vi "main.vi"() -> ()   [LabVIEW 2017]
uses:
  AEROTECstageAPI/SingleStageData.ctl
  AEROTECstageAPI/StageEnum.ctl
  AEROTECstageAPI/MoveDistanceInAxis.ctl
panel:
  in  "Disable Stage":bool
  in  "Distance (mm)":dbl
  in  "Left Button":bool
  in  "Right Button":bool
  in  "Down Button":bool
  in  "Up Button":bool
  in  "Enable Stage":bool
  out "Stage Data":T1[](array[typedef])
  out "error out":errorcluster
  in  "stop 2":bool
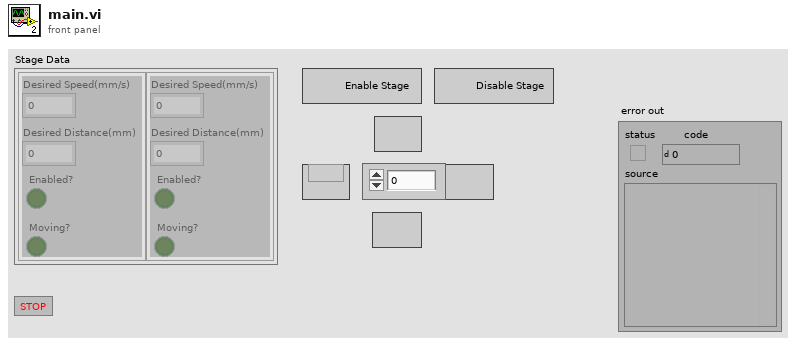
[diagram p1: front panel]
types:
  T1 = typedef "SingleStageData.ctl" = cluster{"Desired Speed(mm/s)":dbl, "Desired Distance(mm)":dbl, "Enabled?":bool, "Moving?":bool}
  T2 = typedef "StageEnum.ctl" = enum16{"Move axis!", "Enable Stage!", "Stop Stage Controller!", "Set Default Speeds!", "Get Stage Parameters", "Start Stage Controller!", "Init"}
  T3 = typedef "MoveDistanceInAxis.ctl" = cluster{"Axis Number":i16, "Distance (mm)":dbl}
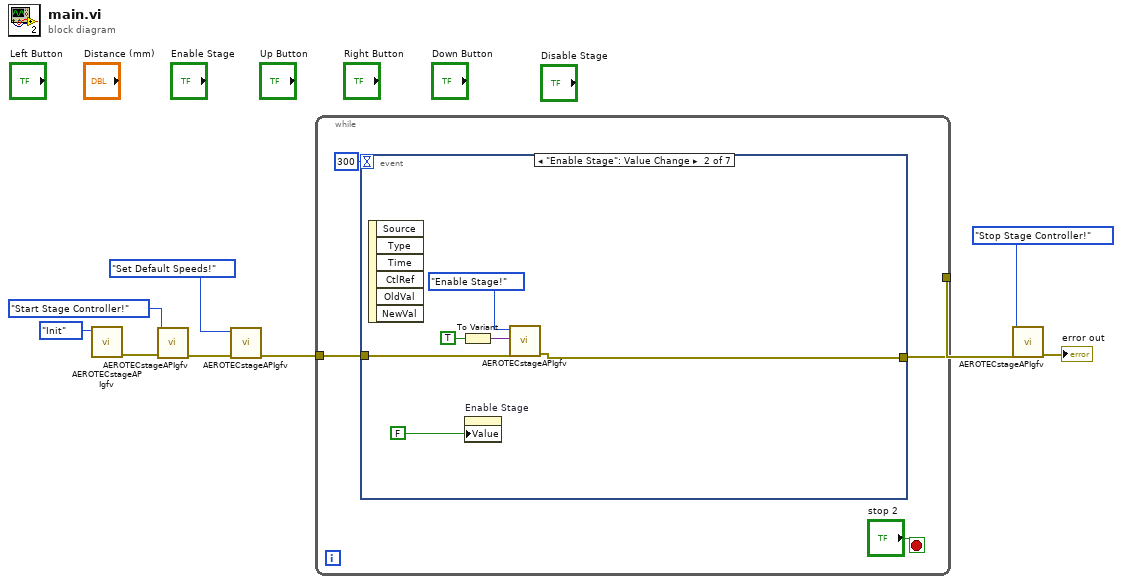
[diagram p0: block diagram]
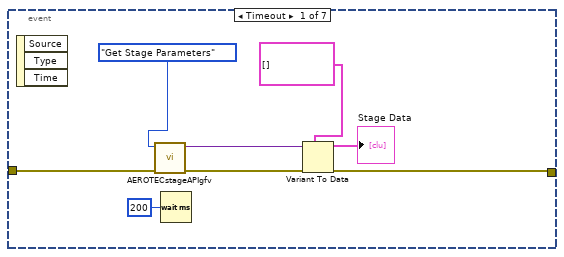
[diagram p2: hidden frame]
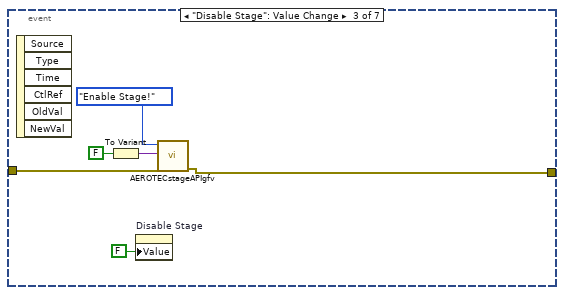
[diagram p3: hidden frame]
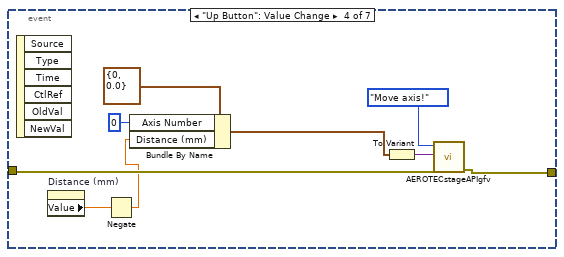
[diagram p4: hidden frame]
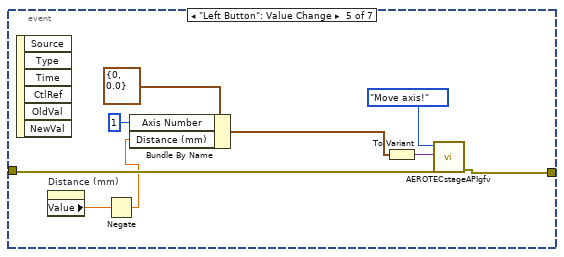
[diagram p5: hidden frame]
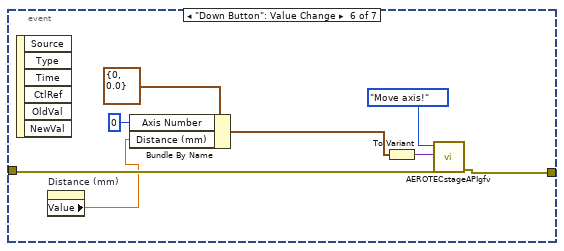
[diagram p6: hidden frame]
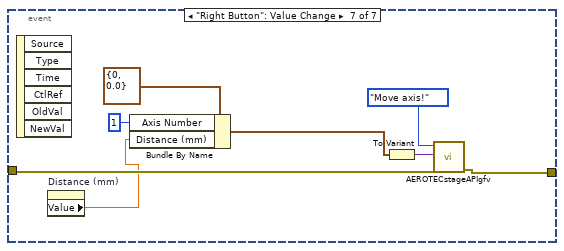
[diagram p7: hidden frame]
diagram:
  n1 = call "AEROTECstageAPIgfv.vi"(11:StageEnum."Init") -> ("error out"=w8:errorcluster)  [unwired: 9 in, 1 out]
  n2 = call "AEROTECstageAPIgfv.vi"("error in (no error)"=w8, 11:StageEnum."Start Stage Controller!") -> ("error out"=w4:errorcluster)  [unwired: 8 in, 1 out]
  n3 = call "AEROTECstageAPIgfv.vi"("error in (no error)"=w4, 11:StageEnum."Set Default Speeds!") -> ("error out"=w2:errorcluster)  [unwired: 8 in, 1 out]
  n4 = while {
    tunnel: w2 -> [w11]
    tunnel: [w10] -> w1
    stop <- "stop 2" stop-if-true
    n5 = event shown="[1] \"Enable Stage\": Value Change" {
      selector: _ -> [_ _ _ _ _ _ _]
      dyn-events: _ -> [_ _ _ _ _ _ _]
      timeout: 300 -> [_ _ _ _ _ _ _]
      tunnel: w11 -> [w16 w26 w32 w41 w50 w58 w66]
      tunnel: [w14 w25 w31 w40 w49 w57 w65] -> w10
      event Timeout {
        n6 = event-data() -> ()  [unwired: 1 in, 3 out]
        n7 = call "AEROTECstageAPIgfv.vi"("error in (no error)"=w16, 11:StageEnum."Get Stage Parameters") -> ("error out"=w14:errorcluster, "Data Out"=w20:variant)  [unwired: 8 in]
        n8 = Wait (ms)(milliseconds to wait=u32 200) -> ()  [unwired: 1 out]
        n9 = Variant To Data(type=T1[] [], Variant=w20) -> (data=→"Stage Data":T1[])  [unwired: 1 in, 1 out]
      }
      event "Enable Stage": Value Change {
        n10 = event-data() -> ()  [unwired: 1 in, 6 out]
        n11 = To Variant(anything=TRUE) -> (Variant=w22:variant)
        n12 = property on="Enable Stage" class="Bool (strict)"("Value"=FALSE) -> ()  [unwired: 2 in, 2 out]
        n13 = call "AEROTECstageAPIgfv.vi"("error in (no error)"=w26, "Data in"=w22, 11:StageEnum."Enable Stage!") -> ("error out"=w25:errorcluster)  [unwired: 7 in, 1 out]
      }
      event "Disable Stage": Value Change {
        n14 = event-data() -> ()  [unwired: 1 in, 6 out]
        n15 = To Variant(anything=FALSE) -> (Variant=w28:variant)
        n16 = property on="Disable Stage" class="Bool (strict)"("Value"=FALSE ("Disable Stage")) -> ()  [unwired: 2 in, 2 out]
        n17 = call "AEROTECstageAPIgfv.vi"("error in (no error)"=w32, "Data in"=w28, 11:StageEnum."Enable Stage!") -> ("error out"=w31:errorcluster)  [unwired: 7 in, 1 out]
      }
      event "Up Button": Value Change {
        n18 = event-data() -> ()  [unwired: 1 in, 6 out]
        n19 = property on="Distance (mm)" class="DigNum (strict)"() -> ("Value"=w34:dbl)  [unwired: 2 in, 2 out]
        n20 = Negate(x=w34) -> (-x=w33:dbl)
        n21 = Bundle By Name(cluster=T3 {"Axis Number"=0, "Distance (mm)"=0.0} ("MoveDistanceInAxis"), "Axis Number"=i16 0, "Distance (mm)"=w33) -> (w35:T3)
        n22 = To Variant(anything=w35) -> (Variant=w38:variant)
        n23 = call "AEROTECstageAPIgfv.vi"("error in (no error)"=w41, "Data in"=w38, 11:StageEnum."Move axis!") -> ("error out"=w40:errorcluster)  [unwired: 7 in, 1 out]
      }
      event "Left Button": Value Change {
        n24 = event-data() -> ()  [unwired: 1 in, 6 out]
        n25 = property on="Distance (mm)" class="DigNum (strict)"() -> ("Value"=w43:dbl)  [unwired: 2 in, 2 out]
        n26 = Negate(x=w43) -> (-x=w42:dbl)
        n27 = Bundle By Name(cluster=T3 {"Axis Number"=0, "Distance (mm)"=0.0} ("MoveDistanceInAxis"), "Axis Number"=i16 1, "Distance (mm)"=w42) -> (w44:T3)
        n28 = To Variant(anything=w44) -> (Variant=w47:variant)
        n29 = call "AEROTECstageAPIgfv.vi"("error in (no error)"=w50, "Data in"=w47, 11:StageEnum."Move axis!") -> ("error out"=w49:errorcluster)  [unwired: 7 in, 1 out]
      }
      event "Down Button": Value Change {
        n30 = event-data() -> ()  [unwired: 1 in, 6 out]
        n31 = property on="Distance (mm)" class="DigNum (strict)"() -> ("Value"=w51:dbl)  [unwired: 2 in, 2 out]
        n32 = Bundle By Name(cluster=T3 {"Axis Number"=0, "Distance (mm)"=0.0} ("MoveDistanceInAxis"), "Axis Number"=i16 0, "Distance (mm)"=w51) -> (w52:T3)
        n33 = To Variant(anything=w52) -> (Variant=w55:variant)
        n34 = call "AEROTECstageAPIgfv.vi"("error in (no error)"=w58, "Data in"=w55, 11:StageEnum."Move axis!") -> ("error out"=w57:errorcluster)  [unwired: 7 in, 1 out]
      }
      event "Right Button": Value Change {
        n35 = event-data() -> ()  [unwired: 1 in, 6 out]
        n36 = property on="Distance (mm)" class="DigNum (strict)"() -> ("Value"=w59:dbl)  [unwired: 2 in, 2 out]
        n37 = Bundle By Name(cluster=T3 {"Axis Number"=0, "Distance (mm)"=0.0} ("MoveDistanceInAxis"), "Axis Number"=i16 1, "Distance (mm)"=w59) -> (w60:T3)
        n38 = To Variant(anything=w60) -> (Variant=w63:variant)
        n39 = call "AEROTECstageAPIgfv.vi"("error in (no error)"=w66, "Data in"=w63, 11:StageEnum."Move axis!") -> ("error out"=w65:errorcluster)  [unwired: 7 in, 1 out]
      }
    }
  }
  n40 = call "AEROTECstageAPIgfv.vi"("error in (no error)"=w1, 11:StageEnum."Stop Stage Controller!") -> ("error out"=→"error out":errorcluster)  [unwired: 8 in, 1 out]
